vi "Write Humidity.Zero.vi"(8 "error in (no error)":errorcluster, 10 "Humidity.Zero":dbl, 11 "HTS221 in":refnum<class "HTS221.lvclass">) -> (0 "error out":errorcluster, 3 "HTS221 out":refnum<class "HTS221.lvclass">)   [LabVIEW 2020, in "HTS221.lvclass"]
uses:
  HTS221.lvclass
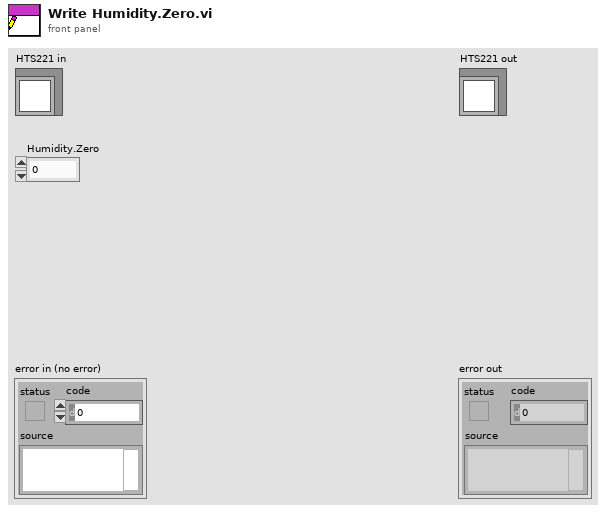
[diagram p1: front panel]
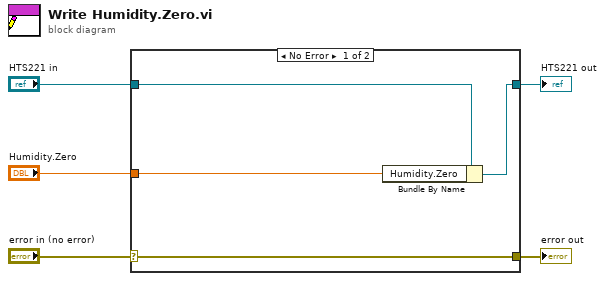
[diagram p0: block diagram]
diagram:
  n1 = case shown="No Error" "error in (no error)" {
    selector: "error in (no error)" -> [w9 w10]
    tunnel: [w9 w10] -> w4
    tunnel: [w7 w11] -> w2
    tunnel: "HTS221 in" -> [w8 w11]
    tunnel: "Humidity.Zero" -> [w6 _]
    frame No Error {
      n2 = Bundle By Name(cluster=w8, "Humidity.Zero"=w6) -> (w7:refnum<class "HTS221.lvclass">)
    }
    frame Error {
    }
  }
  "error out" <- w4
  "HTS221 out" <- w2
